vi "Dialog Play Info.vi"(0 "Enable":bool=TRUE, 5 "error in (no error)":errorcluster) -> (16 "Play Description ind":string caption="Play Description", 17 "Play Name ind":string caption="Play Name", 18 "OK ind":bool caption="OK", 19 "error out":errorcluster)   [LabVIEW 2015]
doc: "Displays a standard dialog box that prompts users to enter information, such as a user name and password.\n--------------------\n\nThis Express VI is configured as follows:\n\nMessage to Display to the User:Please enter a name for this Play, do not include a file type.\nThe inputs are: \nText Entry Box: Play Name\nText Entry Box: Play Description"
uses:
  <vilib>/Utility/miscctls.llb/LVPointTypeDef.ctl
panel:
  out "String 2":string="Enter a description for this play, make it concise." caption="String"
  in  "Play Description":string
  in  "Play Name":string
  out "String":string="Please enter a name for this Play, do not include a file type."
  in  "Cancel":bool
  in  "OK2":bool
  in  "OK1":bool
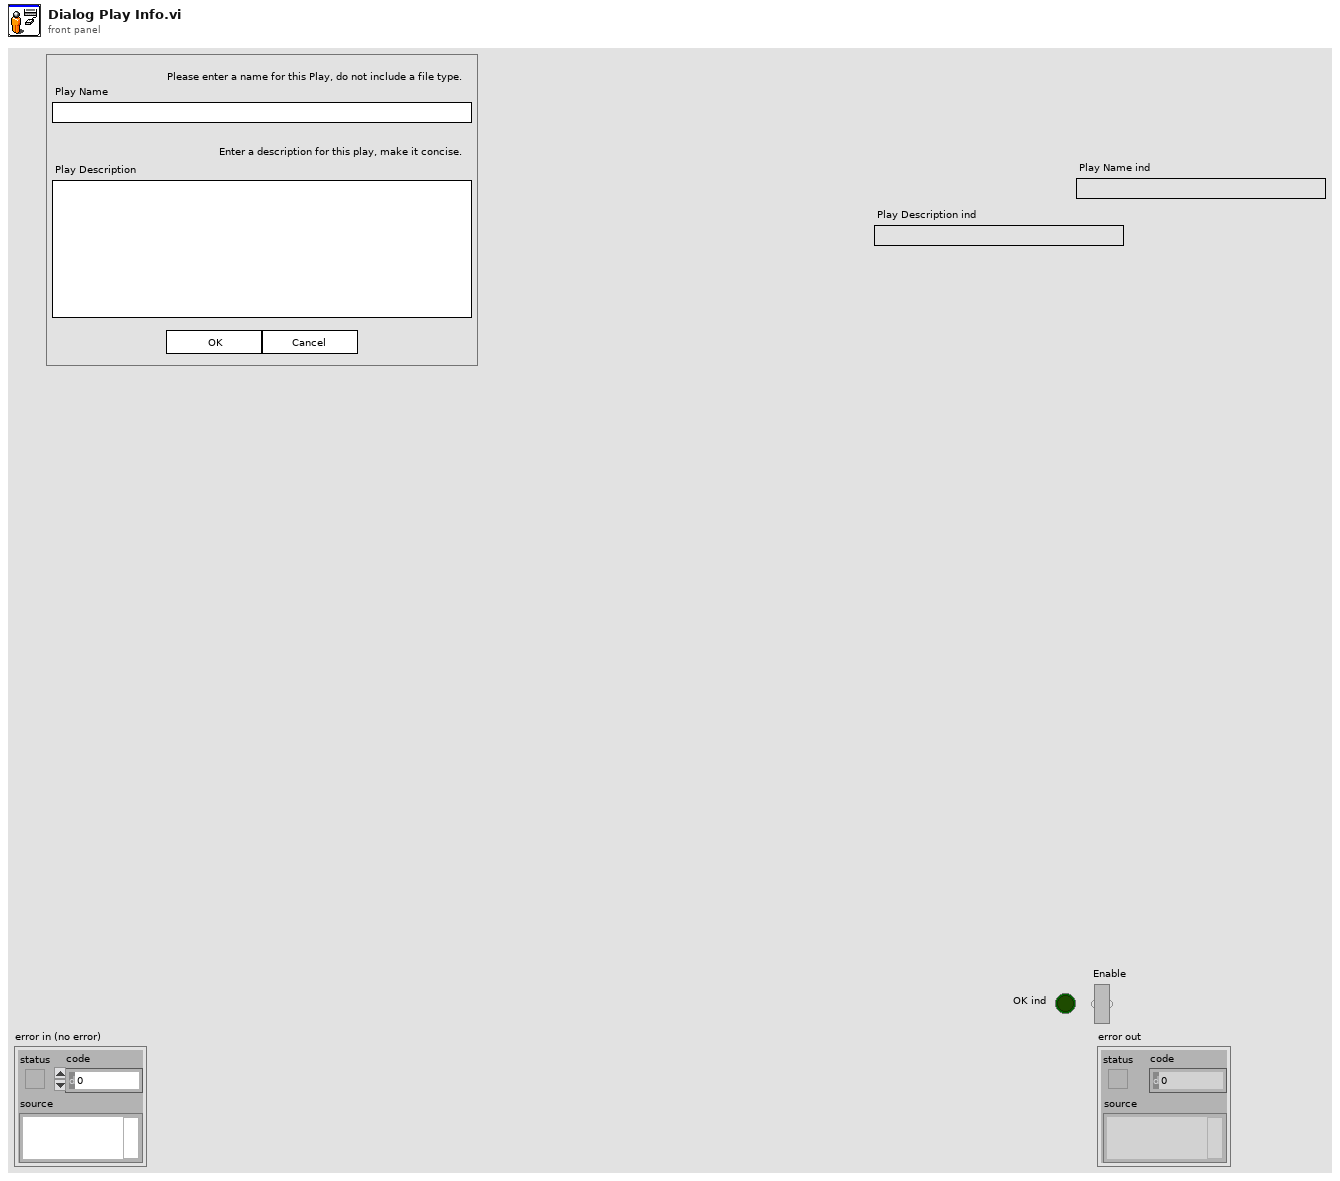
[diagram p1: front panel]
types:
  T1 = typedef "LVPointTypeDef.ctl" = cluster{"Horizontal":i16, "Vertical":i16}
  T2 = cluster{"Input Name":string, "Input Data Type":i32}[]
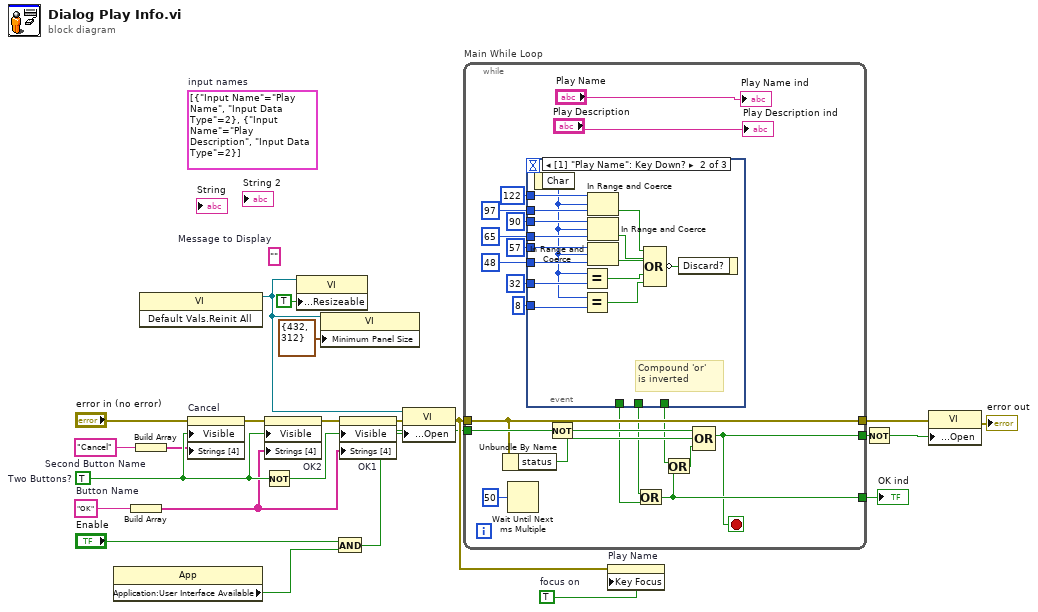
[diagram p0: block diagram]
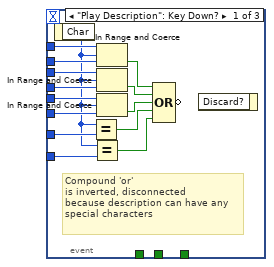
[diagram p2: hidden frame]
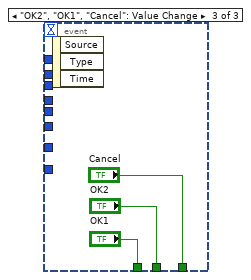
[diagram p3: hidden frame]
diagram:
  w5 = TRUE  # focus on
  (unwired) T2 [{"Input Name"="Play Name", "Input Data Type"=2}, {"Input Name"="Play Description", "Input Data Type"=2}]  # input names
  w16 = "Cancel"  # Second Button Name
  w14 = "OK"  # Button Name
  (unwired) ""  # Message to Display
  w23 = TRUE  # Two Buttons?
  n1 = property class="App"() -> ("Application:User Interface Available"=w6:bool)  [unwired: 2 in, 2 out]
  n2 = Build Array(w14) -> (w15:string[])
  n3 = Build Array(w16) -> (w17:string[])
  n4 = invoke class="VI" method="Default Vals.Reinit All"() -> (reference out=w4:refnum<vi>)  [unwired: 3 in, 2 out]
  n5 = property on="Cancel" class="Bool"(error in="error in (no error)", "Visible"=w23, "Strings [4]"=w17) -> (error out=w20:errorcluster)  [unwired: 1 in, 1 out]
  n6 = Not(x=w23) -> (.not. x?=w21:bool)
  n7 = property on="OK2" class="Bool"(error in=w20, "Visible"=w23, "Strings [4]"=w15) -> (error out=w19:errorcluster)  [unwired: 1 in, 1 out]
  n8 = property class="VI"(reference=w4, "Front Panel.Resizeable"=TRUE ("Front Panel Window:Resizable")) -> ()  [unwired: 1 in, 2 out]
  n9 = property class="VI"(reference=w4, "Minimum Panel Size"=T1 {"Horizontal"=432, "Vertical"=312} ("Front Panel Window:Minimum Size")) -> ()  [unwired: 1 in, 2 out]
  n10 = And(x="Enable", y=w6) -> (x .and. y?=w7:bool)
  n11 = property on="OK1" class="Bool"(error in=w19, "Visible"=w21, "Strings [4]"=w15) -> (error out=w13:errorcluster)  [unwired: 1 in, 1 out]
  n12 = property class="VI"(reference=w4, error in=w13, "Front Panel Window:Open"=w7) -> (error out=w12:errorcluster)  [unwired: 1 out]
  n13 = while "Main While Loop" {
    tunnel: [w43] -> w22
    tunnel: w7 -> [w42]
    tunnel: [w40] -> w18
    tunnel: w12 -> [w39]
    tunnel: [w39] -> w10
    stop <- w40 stop-if-true
    n14 = Unbundle By Name(w39) -> ("status"=w37:bool)
    n15 = Wait Until Next ms Multiple(millisecond multiple=u32 50) -> ()  [unwired: 1 out]
    n16 = event shown="[1] \"Play Name\": Key Down?" {
      selector: _ -> [_ _ _]
      dyn-events: _ -> [_ _ _]
      timeout: _ -> [_ _ _]
      tunnel: [_ _ "Cancel"] -> w36
      tunnel: [_ _ "OK2"] -> w35
      tunnel: [_ _ "OK1"] -> w34
      tunnel: i16 32 -> [w54 w62 _]
      tunnel: i16 48 -> [w53 w63 _]
      tunnel: i16 57 -> [w52 w64 _]
      tunnel: i16 65 -> [w51 w65 _]
      tunnel: i16 90 -> [w50 w66 _]
      tunnel: i16 97 -> [w49 w67 _]
      tunnel: i16 122 -> [w48 w68 _]
      tunnel: i16 8 -> [w45 w59 _]
      event "Play Description": Key Down? {
        # "Compound 'or' \nis inverted, disconnected\nbecause description can have any\nspecial characters"
        n17 = event-data() -> ("Char"=w46:i16)  [unwired: 1 in]
        n18 = Equal?(x=w46, y=w54) -> (x = y?=w58:bool)
        n19 = Equal?(x=w46, y=w45) -> (x = y?=w47:bool)
        n20 = In Range and Coerce(upper limit=w48, x=w46, lower limit=w49) -> (In Range?=w55:bool)  [unwired: 1 out]
        n21 = In Range and Coerce(upper limit=w50, x=w46, lower limit=w51) -> (In Range?=w56:bool)  [unwired: 1 out]
        n22 = In Range and Coerce(upper limit=w52, x=w46, lower limit=w53) -> (In Range?=w57:bool)  [unwired: 1 out]
        n23 = Compound Arithmetic op=OR(w55, w56, w57, w58, w47) -> ()  [unwired: 1 out]
        n24 = event-data() -> ()  [unwired: 2 in, 1 out]
      }
      event "Play Name": Key Down? {
        # "Compound 'or' \nis inverted"
        n25 = event-data() -> ("Char"=w61:i16)  [unwired: 1 in]
        n26 = Equal?(x=w61, y=w62) -> (x = y?=w73:bool)
        n27 = Equal?(x=w61, y=w59) -> (x = y?=w60:bool)
        n28 = In Range and Coerce(upper limit=w68, x=w61, lower limit=w67) -> (In Range?=w70:bool)  [unwired: 1 out]
        n29 = In Range and Coerce(upper limit=w66, x=w61, lower limit=w65) -> (In Range?=w71:bool)  [unwired: 1 out]
        n30 = In Range and Coerce(upper limit=w64, x=w61, lower limit=w63) -> (In Range?=w72:bool)  [unwired: 1 out]
        n31 = Compound Arithmetic op=OR(w70, w71, w72, w73, w60) -> (invert w69:bool)
        n32 = event-data("Discard?"=w69) -> ()  [unwired: 1 in, 1 out]
      }
      event "OK2", "OK1", "Cancel": Value Change {
        n33 = event-data() -> ()  [unwired: 1 in, 3 out]
      }
    }
    n34 = Not(x=w42) -> (.not. x?=w41:bool)
    n35 = Or(x=w35, y=w34) -> (x .or. y?=w43:bool)
    n36 = Or(x=w36, y=w43) -> (x .or. y?=w38:bool)
    n37 = Compound Arithmetic op=OR(w41, w37, w38) -> (w40:bool)
    "Play Description ind" <- "Play Description"
    "Play Name ind" <- "Play Name"
  }
  "OK ind" <- w22
  n38 = property on="Play Name" class="Str"(error in=w12, "Key Focus"=w5) -> ()  [unwired: 1 in, 2 out]
  n39 = Not(x=w18) -> (.not. x?=w1:bool)
  n40 = property class="VI"(error in=w10, "Front Panel Window:Open"=w1) -> (error out=→"error out":errorcluster)  [unwired: 1 in, 1 out]
